vi "wash needle.vi"   [LabVIEW 2023]
types:
  T1 = enum16{"plate1", "plate2", "plate3", "rinse", "seat"}
  T2 = enum16{"Initialize", "Absolute Position", "Relative Pickup", "Relative Dispense", "Swich valve", "Bypass"}
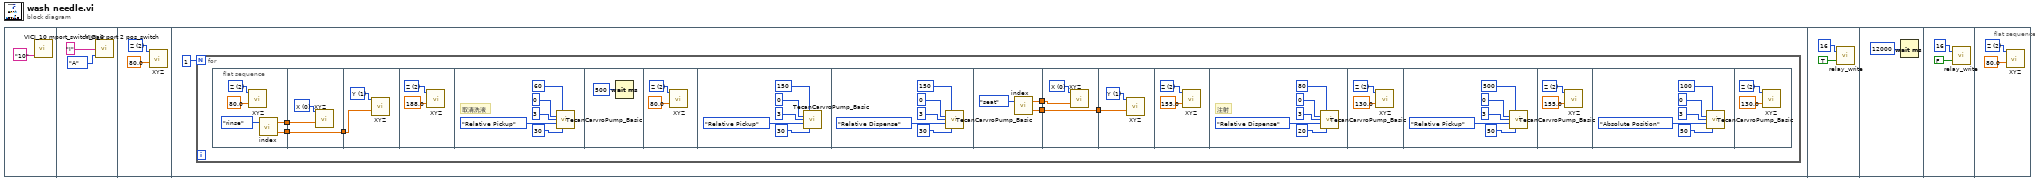
[diagram p0: block diagram]
diagram:
  n1 = flat-sequence {
    frame #0 {
      n2 = call "VICI_10 mport_switch_pair.vi"("Go to position"="10") -> ()  [unwired: 3 in, 1 out]
    }
    frame #1 {
      n3 = call "VICI_6 port 2 pos_switch.vi"("Switch to position (A/B)"=enum16{"A", "B"}."A", "Valve ID"="I") -> ()  [unwired: 2 in, 1 out]
    }
    frame #2 {
      w5 = u16 2 items=["X", "Y", "Z"] ("AXIS")
      n4 = call "XYZ.vi"("AXIS"=w5, "Set location (mm)"=80.0) -> ()  [unwired: 9 in, 5 out]
    }
    frame #3 {
      n5 = for {
        N: 1 -> [_]
        n6 = flat-sequence {
          tunnel: [w14] -> w12
          tunnel: [w13] -> w10
          tunnel: w12 -> [w19]
          tunnel: [w18] -> w11
          tunnel: w10 -> [w18]
          tunnel: w11 -> [w21]
          tunnel: [w44] -> w9
          tunnel: [w43] -> w7
          tunnel: w9 -> [w47]
          tunnel: [w46] -> w8
          tunnel: w7 -> [w46]
          tunnel: w8 -> [w49]
          frame #0 {
            w17 = u16 2 items=["X", "Y", "Z"] ("AXIS")
            n7 = call "XYZ.vi"("AXIS"=w17, "Set location (mm)"=80.0) -> ()  [unwired: 9 in, 5 out]
            n8 = call "index.vi"("where"=T1."rinse") -> ("Y"=w13:dbl, "X"=w14:dbl)  [unwired: 1 in]
          }
          frame #1 {
            w20 = u16 0 items=["X", "Y", "Z"] ("AXIS")
            n9 = call "XYZ.vi"("AXIS"=w20, "Set location (mm)"=w19) -> ()  [unwired: 9 in, 5 out]
          }
          frame #2 {
            w22 = u16 1 items=["X", "Y", "Z"] ("AXIS")
            n10 = call "XYZ.vi"("AXIS"=w22, "Set location (mm)"=w21) -> ()  [unwired: 9 in, 5 out]
          }
          frame #3 {
            w24 = u16 2 items=["X", "Y", "Z"] ("AXIS")
            n11 = call "XYZ.vi"("AXIS"=w24, "Set location (mm)"=188.0) -> ()  [unwired: 9 in, 5 out]
          }
          frame #4 {
            # "取清洗液"
            n12 = call "TecanCarvroPump_Basic.vi"("Volume (μL)"=u16 60, "TecanPump address"=u8 0, "Valve"=u8 3, "Mode"=T2."Relative Pickup", "Speed (μL/s)"=u16 30) -> ()  [unwired: 10 in, 1 out]
          }
          frame #5 {
            n13 = Wait (ms)(milliseconds to wait=u32 500) -> ()  [unwired: 1 out]
          }
          frame #6 {
            w32 = u16 2 items=["X", "Y", "Z"] ("AXIS")
            n14 = call "XYZ.vi"("AXIS"=w32, "Set location (mm)"=80.0) -> ()  [unwired: 9 in, 5 out]
          }
          frame #7 {
            n15 = call "TecanCarvroPump_Basic.vi"("Volume (μL)"=u16 150, "TecanPump address"=u8 0, "Valve"=u8 3, "Mode"=T2."Relative Pickup", "Speed (μL/s)"=u16 30) -> ()  [unwired: 10 in, 1 out]
          }
          frame #8 {
            n16 = call "TecanCarvroPump_Basic.vi"("Volume (μL)"=u16 150, "TecanPump address"=u8 0, "Valve"=u8 3, "Mode"=T2."Relative Dispense", "Speed (μL/s)"=u16 30) -> ()  [unwired: 10 in, 1 out]
          }
          frame #9 {
            n17 = call "index.vi"("where"=T1."seat") -> ("Y"=w43:dbl, "X"=w44:dbl)  [unwired: 1 in]
          }
          frame #10 {
            w48 = u16 0 items=["X", "Y", "Z"] ("AXIS")
            n18 = call "XYZ.vi"("AXIS"=w48, "Set location (mm)"=w47) -> ()  [unwired: 9 in, 5 out]
          }
          frame #11 {
            w50 = u16 1 items=["X", "Y", "Z"] ("AXIS")
            n19 = call "XYZ.vi"("AXIS"=w50, "Set location (mm)"=w49) -> ()  [unwired: 9 in, 5 out]
          }
          frame #12 {
            w52 = u16 2 items=["X", "Y", "Z"] ("AXIS")
            n20 = call "XYZ.vi"("AXIS"=w52, "Set location (mm)"=155.0) -> ()  [unwired: 9 in, 5 out]
          }
          frame #13 {
            # "注射"
            n21 = call "TecanCarvroPump_Basic.vi"("Volume (μL)"=u16 80, "TecanPump address"=u8 0, "Valve"=u8 3, "Mode"=T2."Relative Dispense", "Speed (μL/s)"=u16 20) -> ()  [unwired: 10 in, 1 out]
          }
          frame #14 {
            w59 = u16 2 items=["X", "Y", "Z"] ("AXIS")
            n22 = call "XYZ.vi"("AXIS"=w59, "Set location (mm)"=130.0) -> ()  [unwired: 9 in, 5 out]
          }
          frame #15 {
            n23 = call "TecanCarvroPump_Basic.vi"("Volume (μL)"=u16 500, "TecanPump address"=u8 0, "Valve"=u8 3, "Mode"=T2."Relative Pickup", "Speed (μL/s)"=u16 50) -> ()  [unwired: 10 in, 1 out]
          }
          frame #16 {
            w65 = u16 2 items=["X", "Y", "Z"] ("AXIS")
            n24 = call "XYZ.vi"("AXIS"=w65, "Set location (mm)"=155.0) -> ()  [unwired: 9 in, 5 out]
          }
          frame #17 {
            n25 = call "TecanCarvroPump_Basic.vi"("Volume (μL)"=u16 100, "TecanPump address"=u8 0, "Valve"=u8 3, "Mode"=T2."Absolute Position", "Speed (μL/s)"=u16 50) -> ()  [unwired: 10 in, 1 out]
          }
          frame #18 {
            w73 = u16 2 items=["X", "Y", "Z"] ("AXIS")
            n26 = call "XYZ.vi"("AXIS"=w73, "Set location (mm)"=130.0) -> ()  [unwired: 9 in, 5 out]
          }
        }
      }
    }
    frame #4 {
      n27 = call "relay_write.vi"("on/off"=TRUE, "No."=u8 16) -> ()  [unwired: 1 out]
    }
    frame #5 {
      n28 = Wait (ms)(milliseconds to wait=u32 12000) -> ()  [unwired: 1 out]
    }
    frame #6 {
      n29 = call "relay_write.vi"("on/off"=FALSE, "No."=u8 16) -> ()  [unwired: 1 out]
    }
    frame #7 {
      w80 = u16 2 items=["X", "Y", "Z"] ("AXIS")
      n30 = call "XYZ.vi"("AXIS"=w80, "Set location (mm)"=80.0) -> ()  [unwired: 9 in, 5 out]
    }
  }
